vi "Readings.vi"() -> ()   [LabVIEW 2020]
panel:
  in  "S3":dbl
  in  "S2":dbl
  in  "S1":dbl
  in  "T3":dbl
  in  "T2":dbl
  in  "T1":dbl
  in  "T0":dbl
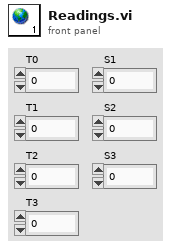
[diagram p1: front panel]
diagram:
